vi "LoadPrograms.vi"(0 "Program Interface in":refnum<class "Program Interface.lvclass">, 5 "error in (no error)":errorcluster) -> (14 "Program Interface out":refnum<class "Program Interface.lvclass">, 19 "error out":errorcluster)   [LabVIEW 2019, in "Program Interface.lvclass"]
uses:
  Program Interface.lvclass
  C:/_Code/Development/Sub-Zero Functional Test/standard hardware/Universal Robots/UR LabVIEW Interface/Classes/Application/Application Interfaces/Application Interface/Application Interface.lvclass
  Program Interface.lvclass/Program Interface.ctl
  Application.lvclass
  Program List/Program List.lvclass
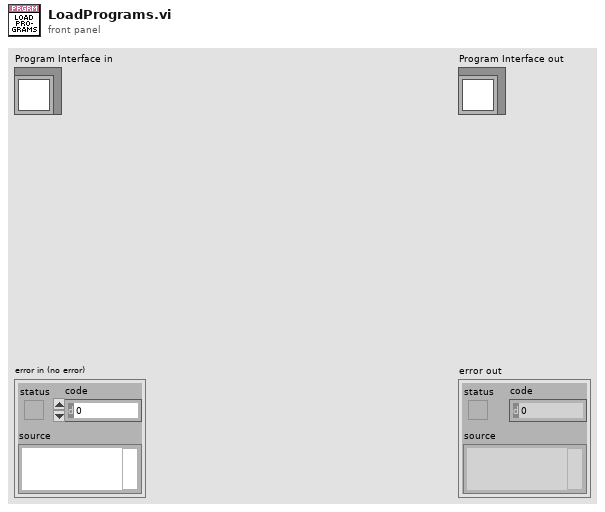
[diagram p1: front panel]
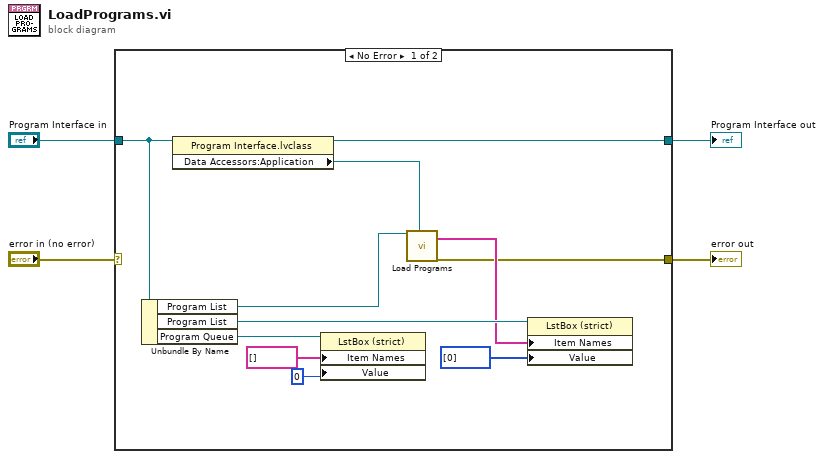
[diagram p0: block diagram]
diagram:
  n1 = case shown="No Error" "error in (no error)" {
    selector: "error in (no error)" -> [_ w17]
    tunnel: [w5 w17] -> w3
    tunnel: [w15 w16] -> w1
    tunnel: "Program Interface in" -> [w14 w16]
    frame No Error {
      n2 = Unbundle By Name(w14) -> ("Program List"=w8:refnum<class "Program List.lvclass">, "Program List"=w13:refnum<vi>, "Program Queue"=w12:refnum<vi>)
      n3 = property class="Program Interface.lvclass"(reference=w14) -> (reference out=w15:refnum<class "Program Interface.lvclass">, "Data Accessors:Application"=w7:refnum<class "Application.lvclass">)  [unwired: 1 in, 1 out]
      n4 = property class="LstBox (strict)"(reference=w12, "Item Names"=string[] [], "Value"=0) -> ()  [unwired: 1 in, 2 out]
      n5 = call-dynamic "Load Programs.vi"("Program List in"=w8, "Application.lvclass"=w7) -> ("Programs"=w6:string[], "error out"=w5:errorcluster)  [unwired: 15 in, 1 out]
      n6 = property class="LstBox (strict)"(reference=w13, "Item Names"=w6, "Value"=i32[] [0]) -> ()  [unwired: 1 in, 2 out]
    }
    frame Error {
    }
  }
  "error out" <- w3
  "Program Interface out" <- w1
